vi "dfd_Draw Delay.vi"(4 "variable":string, 5 "fonts input":T1(array[cluster]), 6 "alignment(left, top)":T2, 7 "equation type":enum16{"Continuous", "Discrete"}(ring), 9 "origin":cluster{"x":i16, "y":i16}, 10 "delay":dbl, 11 "picture":picture) -> (1 "text rect":T3, 3 "new picture":picture)   [LabVIEW 2017, in "NI_DigFilter_Process.lvlib"]
uses:
  <vilib>/addons/Digital Filter Design/NI_DigFilter_Process.lvlib
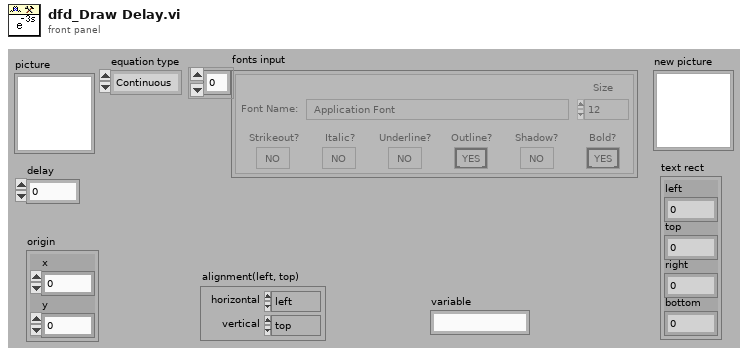
[diagram p1: front panel]
types:
  T1 = cluster{"Font Name:":string, "Size":i16, "Strikeout?":bool, "Italic?":bool, "Underline?":bool, "Outline?":bool, "Shadow?":bool, "Bold?":bool}[]
  T2 = cluster{"horizontal":enum16{"left", "center", "right"}, "vertical":enum16{"top", "center", "bottom"}}
  T3 = cluster{"left":i16, "top":i16, "right":i16, "bottom":i16}
  T4 = enum16{"User-specified Font", "Application Font", "System Font", "Dialog Font"}
  T5 = cluster{"Font Name:":string, "Size":i16, "Strikeout?":bool, "Italic?":bool, "Underline?":bool, "Outline?":bool, "Shadow?":bool, "Bold?":bool}
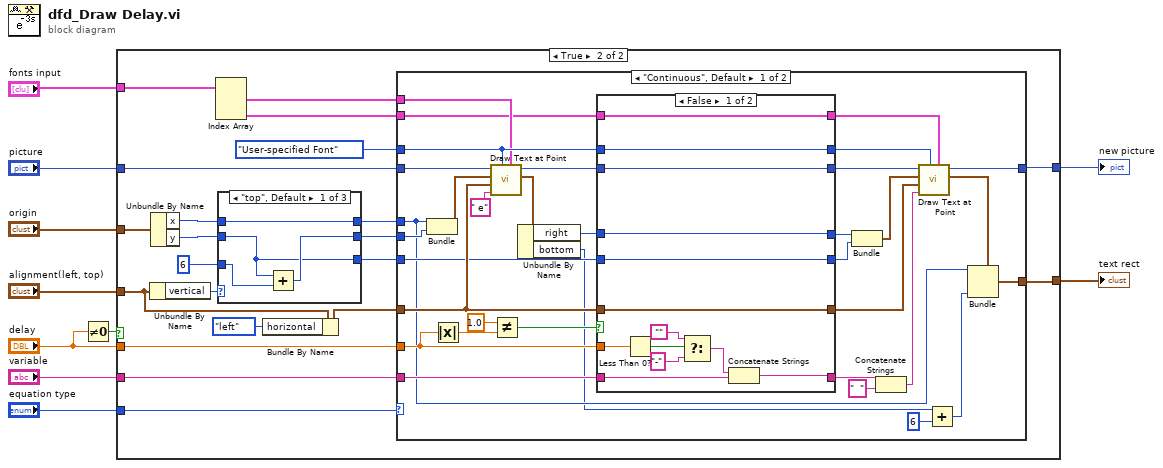
[diagram p0: block diagram]
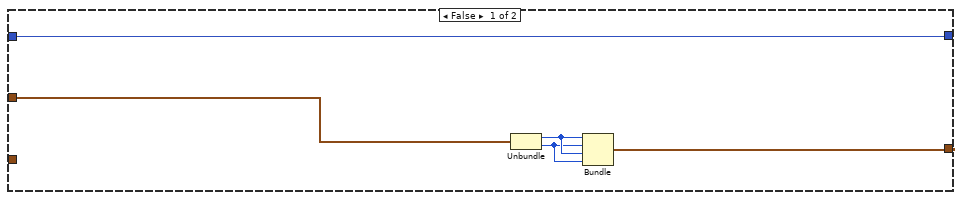
[diagram p2: hidden frame]
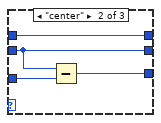
[diagram p3: hidden frame]
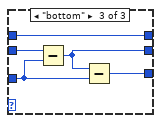
[diagram p4: hidden frame]
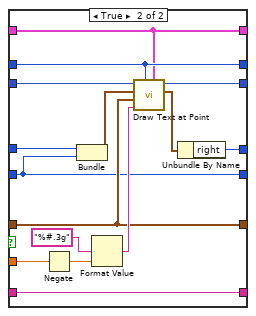
[diagram p5: hidden frame]
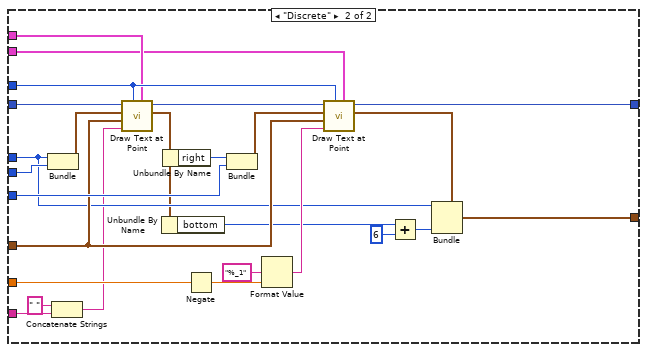
[diagram p6: hidden frame]
diagram:
  n1 = Not Equal To 0?(x="delay") -> (x != 0?=w4:bool)
  n2 = case shown="True" w4 {
    tunnel: "picture" -> [w11 w36]
    tunnel: "origin" -> [w13 w29]
    tunnel: "delay" -> [_ w35]
    tunnel: "variable" -> [_ w34]
    tunnel: "equation type" -> [_ w33]
    tunnel: [w12 w16] -> w6
    tunnel: [w11 w31] -> w5
    tunnel: "fonts input" -> [_ w24]
    tunnel: "alignment(left, top)" -> [_ w19]
    frame False {
      n3 = Unbundle(w13) -> ("x"=w15:i16, "y"=w14:i16)
      n4 = Bundle("x"=w15, "y"=w14, "x"=w15, "y"=w14) -> (w12:cluster{"x":i16, "y":i16, "x":i16, "y":i16})  [unwired: 1 out]
    }
    frame True {
      n5 = Unbundle By Name(w19) -> ("vertical"=w30:enum16{"top", "center", "bottom"})
      n6 = Unbundle By Name(w29) -> ("x"=w28:i16, "y"=w26:i16)
      n7 = Index Array(array=w24) -> (element #1=w23:T5, element #3=w22:T5)  [unwired: 3 in, 1 out]
      n8 = case shown="\"top\", Default" w30 {
        tunnel: w28 -> [w40 w44 w49]
        tunnel: [w40 w44 w49] -> w21
        tunnel: w26 -> [w37 w42 w48]
        tunnel: i16 6 ("y") -> [w39 w43 w46]
        tunnel: [w38 w42 w47] -> w20
        tunnel: [w37 w41 w45] -> w18
        frame "top", Default {
          n9 = Add(x=w37, y=w39) -> (x+y=w38:i16)
        }
        frame "center" {
          n10 = Subtract(x=w42, y=w43) -> (x-y=w41:i16)
        }
        frame "bottom" {
          n11 = Subtract(x=w48, y=w46) -> (x-y=w47:i16)
          n12 = Subtract(x=w47, y=w46) -> (x-y=w45:i16)
        }
      }
      n13 = Bundle By Name(cluster=w19, "horizontal"=enum16{"left", "center", "right"}."left") -> (w17:T2)
      n14 = case shown="\"Continuous\", Default" w33 {
        tunnel: w35 -> [w79 w135]
        tunnel: w36 -> [w83 w137]
        tunnel: w34 -> [w82 w114]
        tunnel: [w81 w136] -> w31
        tunnel: [w80 w127] -> w16
        tunnel: T4."User-specified Font" ("desired font(Application)") -> [w78 w134]
        tunnel: w23 -> [w67 w125]
        tunnel: w22 -> [w66 w122]
        tunnel: w21 -> [w53 w119]
        tunnel: w20 -> [w64 w124]
        tunnel: w17 -> [w65 w120]
        tunnel: w18 -> [w57 w121]
        frame "Continuous", Default {
          n15 = Bundle("x"=w53, "y"=w64) -> (w63:cluster{"x":i16, "y":i16})  [unwired: 1 out]
          n16 = Absolute Value(x=w79) -> (abs(x)=w70:dbl)
          n17 = call <vilib>:"Draw Text at Point.vi"("[user-specified font]"=w67, "desired font(Application)"=w78, "text"=" e", "alignment(left, top)"=w65, "origin"=w63, "picture"=w83) -> ("text rect"=w59:T3, "new picture"=w76:picture)  [unwired: 3 in, 1 out]
          n18 = Not Equal?(x=1.0 ("y"), y=w70) -> (x != y?=w72:bool)
          n19 = Unbundle By Name(w59) -> ("right"=w58:i16, "bottom"=w52:i16)
          n20 = case shown="False" w72 {
            tunnel: w79 -> [w94 w111]
            tunnel: w76 -> [w96 w109]
            tunnel: [w96 w107] -> w75
            tunnel: w65 -> [w95 w106]
            tunnel: [w85 w98] -> w73
            tunnel: [w95 w106] -> w74
            tunnel: w82 -> [w89 w102]
            tunnel: [w91 w102] -> w60
            tunnel: w66 -> [w92 w103]
            tunnel: w78 -> [w93 w104]
            tunnel: [w93 w104] -> w69
            tunnel: [w92 w103] -> w68
            tunnel: w58 -> [w85 w101]
            tunnel: w57 -> [w84 w97]
            tunnel: [w84 w97] -> w56
            frame False {
              n21 = Less Than 0?(x=w94) -> (x < 0?=w90:bool)
              n22 = Select(t="", s=w90, f="-" ("string")) -> (s? t:f=w88:string)
              n23 = Concatenate Strings(w88, w89) -> (w91:string)
            }
            frame True {
              n24 = Negate(x=w111) -> (-x=w105:dbl)
              n25 = Bundle("right"=w101, "y"=w97) -> (w100:cluster{"right":i16, "y":i16})  [unwired: 1 out]
              n26 = Format Value(format string="%#.3g", value (0)=w105) -> (output string=w108:string)  [unwired: 1 out]
              n27 = call <vilib>:"Draw Text at Point.vi"("[user-specified font]"=w103, "desired font(Application)"=w104, "text"=w108, "alignment(left, top)"=w106, "origin"=w100, "picture"=w109) -> ("text rect"=w99:T3, "new picture"=w107:picture)  [unwired: 3 in, 1 out]
              n28 = Unbundle By Name(w99) -> ("right"=w98:i16)
            }
          }
          n29 = Bundle("right"=w73, "y"=w56) -> (w55:cluster{"right":i16, "y":i16})  [unwired: 1 out]
          n30 = Concatenate Strings(w60, "  " ("string")) -> (w61:string)
          n31 = call <vilib>:"Draw Text at Point.vi"("[user-specified font]"=w68, "desired font(Application)"=w69, "text"=w61, "alignment(left, top)"=w74, "origin"=w55, "picture"=w75) -> ("text rect"=w54:T3, "new picture"=w81:picture)  [unwired: 3 in, 1 out]
          n32 = Add(x=w52, y=i16 6) -> (x+y=w50:i16)
          n33 = Bundle(cluster=w54, "left"=w53, "bottom"=w50) -> (w80:T3)  [unwired: 2 out]
        }
        frame "Discrete" {
          n34 = Bundle("x"=w119, "y"=w124) -> (w123:cluster{"x":i16, "y":i16})  [unwired: 1 out]
          n35 = Concatenate Strings(" " ("string"), w114) -> (w113:string)
          n36 = call <vilib>:"Draw Text at Point.vi"("[user-specified font]"=w125, "desired font(Application)"=w134, "text"=w113, "alignment(left, top)"=w120, "origin"=w123, "picture"=w137) -> ("text rect"=w118:T3, "new picture"=w129:picture)  [unwired: 3 in, 1 out]
          n37 = Unbundle By Name(w118) -> ("bottom"=w116:i16)
          n38 = Unbundle By Name(w118) -> ("right"=w128:i16)
          n39 = Negate(x=w135) -> (-x=w132:dbl)
          n40 = Bundle("right"=w128, "y"=w121) -> (w131:cluster{"right":i16, "y":i16})  [unwired: 1 out]
          n41 = Format Value(format string="%_1", value (0)=w132) -> (output string=w130:string)  [unwired: 1 out]
          n42 = call <vilib>:"Draw Text at Point.vi"("[user-specified font]"=w122, "desired font(Application)"=w134, "text"=w130, "alignment(left, top)"=w120, "origin"=w131, "picture"=w129) -> ("text rect"=w126:T3, "new picture"=w136:picture)  [unwired: 3 in, 1 out]
          n43 = Add(x=w116, y=i16 6) -> (x+y=w115:i16)
          n44 = Bundle(cluster=w126, "left"=w119, "bottom"=w115) -> (w127:T3)  [unwired: 2 out]
        }
      }
    }
  }
  "new picture" <- w5
  "text rect" <- w6
